vi "Name_StepPause.vi"() -> (1 "StepPause":string="StepIndex")   [LabVIEW 2016, in "SeqProcessor.lvlib"]
uses:
  SeqProcessor.lvlib
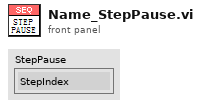
[diagram p1: front panel]
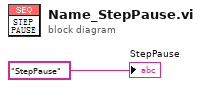
[diagram p0: block diagram]
diagram:
  "StepPause" <- "StepPause" ("Tag")
